vi "DeleteEntry.vi"(3 "error in (no error)":errorcluster, 5 "LotData in":refnum<class "LotData.lvclass">) -> (0 "error out":errorcluster, 1 "DB Message":string, 2 "LotData out":refnum<class "LotData.lvclass">)   [LabVIEW 2012, in "LotData.lvclass"]
uses:
  LotData.lvclass
  <vilib>/addons/database/Auxilliary.llb/DB Tools Parameter Info.ctl
  <vilib>/addons/database/Auxilliary.llb/DB Tools DataTypes.ctl
  <vilib>/addons/database/Auxilliary.llb/DB Tools Parameter Dir.ctl
  LotData.lvclass/LotData.ctl
  <vilib>/addons/database/Connection.llb/DB Tools Open Connec (Path).vi
  <vilib>/addons/database/Command.llb/Cmd Set Parameter Value (C).vi
  <vilib>/addons/database/Command.llb/Cmd Execute.vi
  <vilib>/addons/database/Recordset.llb/Rec Destroy - Command.vi
  <vilib>/addons/database/Command.llb/Cmd Delete.vi
  <vilib>/addons/database/NI_Database_API.lvlib
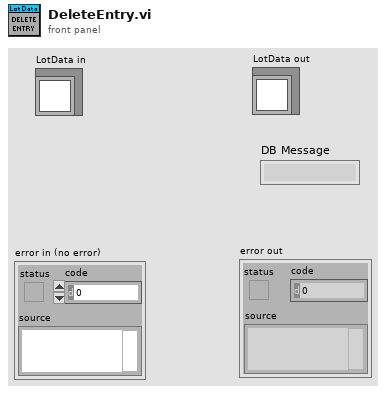
[diagram p1: front panel]
types:
  T1 = typedef "NI_Database_API.lvlib/DB Tools Parameter Info.ctl" = cluster{"parameter name":string, "type":T2, "direction":T3, "value":variant}
  T2 = typedef "NI_Database_API.lvlib/DB Tools DataTypes.ctl" = enum16{"String", "Long (I32)", "Single (SGL)", "Double (DBL)", "Date/Time", "Binary"}
  T3 = typedef "NI_Database_API.lvlib/DB Tools Parameter Dir.ctl" = enum32{"Input", "Output", "Input/Output", "Return Value"}
  T4 = typedef "NI_Database_API.lvlib/Conn ObjectReference.ctl" = refnum<k1>
  T5 = typedef "NI_Database_API.lvlib/Cmd ObjectReference.ctl" = refnum<k1>
  T6 = typedef "NI_Database_API.lvlib/Cmd-Rec Object Reference.ctl" = refnum<k1>
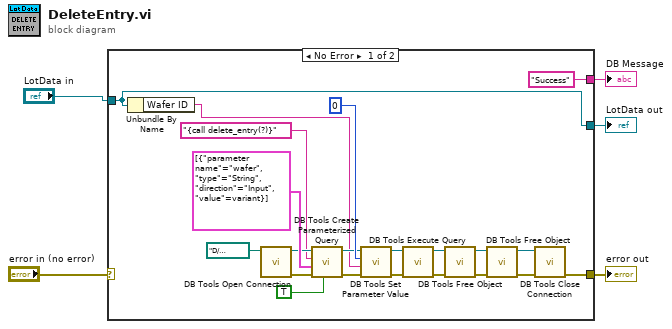
[diagram p0: block diagram]
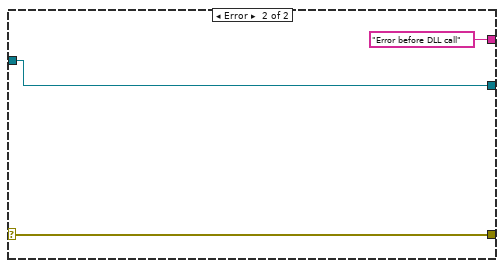
[diagram p2: hidden frame]
diagram:
  n1 = case shown="No Error" "error in (no error)" {
    selector: "error in (no error)" -> [_ w29]
    tunnel: [w7 w29] -> w4
    tunnel: [w26 w28] -> w2
    tunnel: "LotData in" -> [w26 w28]
    tunnel: ["Success" ("DeleteEntry") "Error before DLL call" ("DeleteEntry")] -> w1
    frame No Error {
      n2 = Unbundle By Name(w26) -> ("Wafer ID"=w8:string)
      n3 = call-poly <vilib>:"DB Tools Open Connection.vi"("connection information"=path "D:/Program Files (x86)/National Instruments/LabVIEW 2012/Database/epiDataLink.udl") -> ("error out"=w21:errorcluster, "connection reference"=w22:T4)  [unwired: 7 in]
      n4 = call <vilib>:"DB Tools Create Parameterized Query.vi"("stored procedure? (F)"=TRUE, "error in (no error)"=w21, "parameters"=T1[] [{"parameter name"="wafer", "type"=enum."String", "direction"=enum."Input", "value"=variant}], "SQL query"="{call delete_entry(?)}", "connection reference"=w22) -> ("error out"=w18:errorcluster, "command reference"=w17:T5)  [unwired: 2 in, 1 out]
      n5 = call-poly <vilib>:"DB Tools Set Parameter Value.vi"("error in (no error)"=w18, "value"=w8, "parameter index"=0, "command reference"=w17) -> ("error out"=w13:errorcluster, "command reference out"=w14:T5)  [unwired: 4 in]
      n6 = call-poly <vilib>:"DB Tools Execute Query.vi"("error in (no error)"=w13, "command reference"=w14) -> ("error out"=w12:errorcluster, "command-recordset reference"=w15:T6)  [unwired: 6 in]
      n7 = call-poly <vilib>:"DB Tools Free Object.vi"("error in (no error)"=w12, "command-recordset reference"=w15) -> ("error out"=w16:errorcluster, "command reference"=w9:T5)  [unwired: 8 in]
      n8 = call-poly <vilib>:"DB Tools Free Object.vi"("error in (no error)"=w16, "command reference"=w9) -> ("error out"=w10:errorcluster, "connection reference"=w11:T4)  [unwired: 8 in]
      n9 = call <vilib>:"DB Tools Close Connection.vi"("error in (no error)"=w10, "connection reference"=w11) -> ("error out"=w7:errorcluster)  [unwired: 5 in]
    }
    frame Error {
    }
  }
  "error out" <- w4
  "LotData out" <- w2
  "DB Message" <- w1
